vi "Find Row.vi"(8 "error in":errorcluster, 9 "Index":i32, 10 "SheetData":refnum<k24>) -> (0 "error out":errorcluster, 2 "Row":refnum<k24>)   [LabVIEW 2021, in "Open Xml.lvlib"]
uses:
  Open Xml.lvlib
  C:/Users/tupp_js/.nuget/packages/documentformat.openxml/3.3.0/lib/net46/DocumentFormat.OpenXml.dll
  D:/git/Open-Xml-LabVIEW/DocumentFormat.OpenXml.Framework.dll
  DocumentFormat.OpenXml.Framework.dll
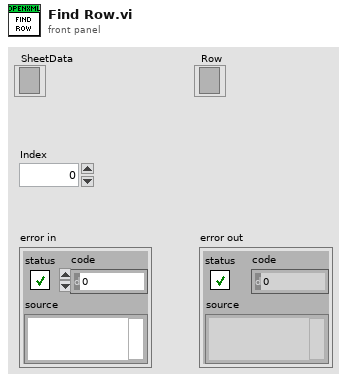
[diagram p1: front panel]
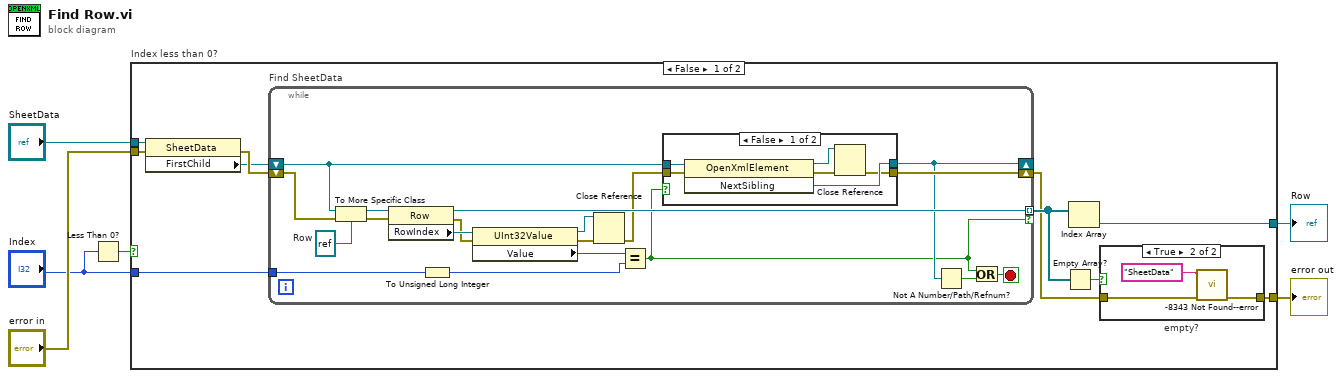
[diagram p0: block diagram]
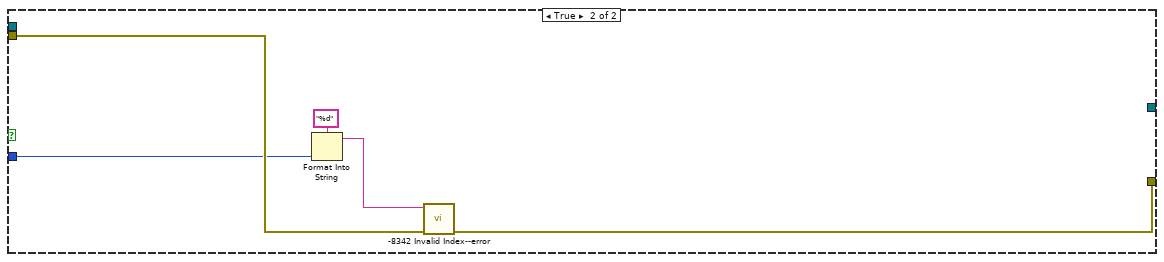
[diagram p4: hidden frame]
diagram:
  n1 = Less Than 0?(x="Index") -> (x < 0?=w3:bool)
  n2 = case "Index less than 0?" shown="False" w3 {
    tunnel: "error in" -> [w14 w52]
    tunnel: "SheetData" -> [w12 _]
    tunnel: "Index" -> [w11 w50]
    tunnel: [w10 _] -> w4
    tunnel: [w7 w51] -> w1
    frame False {
      n3 = property class="SheetData"(reference=w12, error in=w14) -> (error out=w16:errorcluster, "FirstChild"=w15:refnum<k24>)  [unwired: 1 out]
      n4 = while "Find SheetData" {
        shift-right: [w27] -> w8
        shift-left: w16 -> [w39]
        shift-right: [w25] -> _
        shift-left: w15 -> [w26]
        tunnel: [w34] -> w13 mode=indexing if=w24
        tunnel: w11 -> [w29]
        stop <- w37 stop-if-true
        w36 = refnum<k24> refnum  # Row
        n5 = To More Specific Class(target class=w36, reference=w26, error in=w39) -> (specific class reference=w35:refnum<k24>, error out=w31:errorcluster)
        n6 = property class="Row"(reference=w35, error in=w31) -> (reference out=w34:refnum<k24>, error out=w32:errorcluster, "RowIndex"=w33:refnum<k24>)
        n7 = To Unsigned Long Integer(number=w29) -> (unsigned 32bit integer=w22:u32)
        n8 = property class="UInt32Value"(reference=w33, error in=w32) -> (reference out=w21:refnum<k24>, error out=w28:errorcluster, "Value"=w30:u32)
        n9 = Close Reference(reference=w21, error in (no error)=w28) -> (error out=w23:errorcluster)
        n10 = Equal?(x=w30, y=w22) -> (x = y?=w24:bool)
        n11 = case shown="False" w24 {
          tunnel: w23 -> [w45 w46]
          tunnel: [w41 w46] -> w27
          tunnel: [w42 w47] -> w25
          tunnel: w26 -> [w43 w47]
          frame False {
            n12 = invoke class="OpenXmlElement" method="NextSibling"(reference=w43, error in=w45) -> (reference out=w40:refnum<k24>, error out=w44:errorcluster, "NextSibling"=w42:refnum<k24>)  [unwired: 1 in]
            n13 = Close Reference(reference=w40, error in (no error)=w44) -> (error out=w41:errorcluster)
          }
          frame True {
          }
        }
        n14 = Not A Number/Path/Refnum?(number/path/refnum=w25) -> (NaN/Path/Refnum?=w38:bool)
        n15 = Or(x=w24, y=w38) -> (x .or. y?=w37:bool)
      }
      n16 = Empty Array?(array=w13) -> (empty?=w9:bool)
      n17 = Index Array(array=w13) -> (element=w10:refnum<k24>)  [unwired: 1 in]
      n18 = case "empty?" shown="True" w9 {
        tunnel: w8 -> [w17 w20]
        tunnel: [w17 w19] -> w7
        frame False {
        }
        frame True {
          n19 = call "-8343 Not Found--error.vi"("error in (no error)"=w20, "Item"="SheetData") -> ("error out"=w19:errorcluster)  [unwired: 9 in]
        }
      }
    }
    frame True {
      n20 = Format Into String(format string="%d", w50) -> (resulting string=w49:string)  [unwired: 2 in, 1 out]
      n21 = call "-8342 Invalid Index--error.vi"("error in"=w52, "Index"=w49) -> ("error out"=w51:errorcluster)  [unwired: 9 in]
    }
  }
  "error out" <- w1
  "Row" <- w4
